vi "Inject.vi"() -> ()   [LabVIEW 2015]
panel:
  in  "Numeric":i32
  in  "Array":dbl[][](array[numeric])
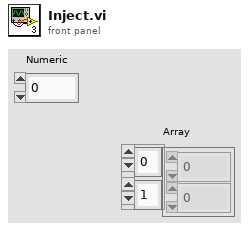
[diagram p1: front panel]
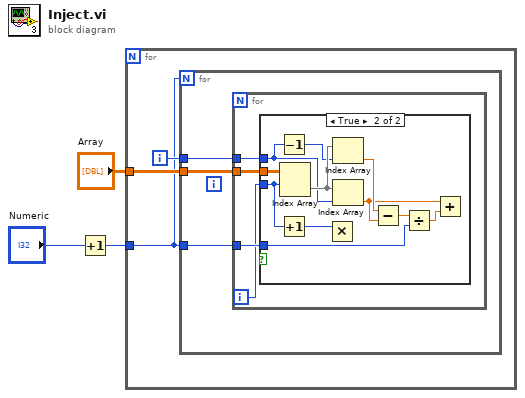
[diagram p0: block diagram]
diagram:
  n1 = Increment(x="Numeric") -> (x+1=w2:i32)
  n2 = for {
    tunnel: "Array" -> [w6]
    tunnel: w2 -> [w4]
    i -> [w5]
    n3 = for {
      N: w4 -> [_]
      tunnel: w6 -> [w9]
      tunnel: w5 -> [w8]
      tunnel: w4 -> [w7]
      n4 = for {
        tunnel: w9 -> [w13]
        tunnel: w8 -> [w12]
        tunnel: w7 -> [w11]
        i -> [w10]
        n5 = case shown="True" {
          selector: _ -> [_ _]
          tunnel: w13 -> [_ w23]
          tunnel: w10 -> [_ w22]
          tunnel: w12 -> [_ w19]
          tunnel: w11 -> [_ w16]
          frame False {
          }
          frame True {
            n6 = Decrement(x=w19) -> (x-1=w18:i32)
            n7 = Increment(x=w22) -> (x+1=w24:i32)
            n8 = Index Array(array=w23, index (row)=w22) -> (element=w21:dbl[])  [unwired: 1 in]
            n9 = Multiply(x=w24) -> ()  [unwired: 1 in, 1 out]
            n10 = Index Array(array=w21, index=w18) -> (element=w20:dbl)
            n11 = Index Array(array=w21, index=w19) -> (element=w14:dbl)
            n12 = Subtract(x=w20, y=w14) -> (x-y=w17:dbl)
            n13 = Divide(x=w17, y=w16) -> (x/y=w15:dbl)
            n14 = Add(x=w14, y=w15) -> ()  [unwired: 1 out]
          }
        }
      }
    }
  }
